vi "2039_hw Brake.vi"(2 "error in (no error)":errorcluster, 3 "CAN Talon SRX Ref":T1[](array[typedef])) -> (0 "error out":errorcluster, 1 "CAN Talon SRX Ref Out":T1[](array[typedef]))   [LabVIEW 2015]
uses:
  <vilib>/Rock Robotics/WPI/MotorControl/WPI_MotorControlDeviceRef.ctl
  <vilib>/Rock Robotics/WPI/MotorControl/WPI_MotorControlType.ctl
  <vilib>/Rock Robotics/SystemInterfaces/DIO/FPGA_DIOPWMChannel.ctl
  <vilib>/Rock Robotics/WPI/PWM/WPI_PWMDeadband.ctl
  <vilib>/Rock Robotics/WPI/CAN/Jaguar/SubVIs/WPI_CANJaguar_ControlMode.ctl
  <vilib>/Rock Robotics/WPI/CAN/TalonSRX/WPI_CANTalonSRX_APIControlMode.ctl
  <vilib>/Rock Robotics/WPI/CAN/TalonSRX/WPI_CANTalonSRX_BrakeOverride.ctl
  <vilib>/Rock Robotics/WPI/Utilities/WPI_GetSetVariantRefNum.vi
  <vilib>/Rock Robotics/WPI/RobotDrive/WPI_RobotDriveMecanumDrive_Cartesian.vi
  <vilib>/Rock Robotics/Network Tables/NT Write Numeric Array.vi
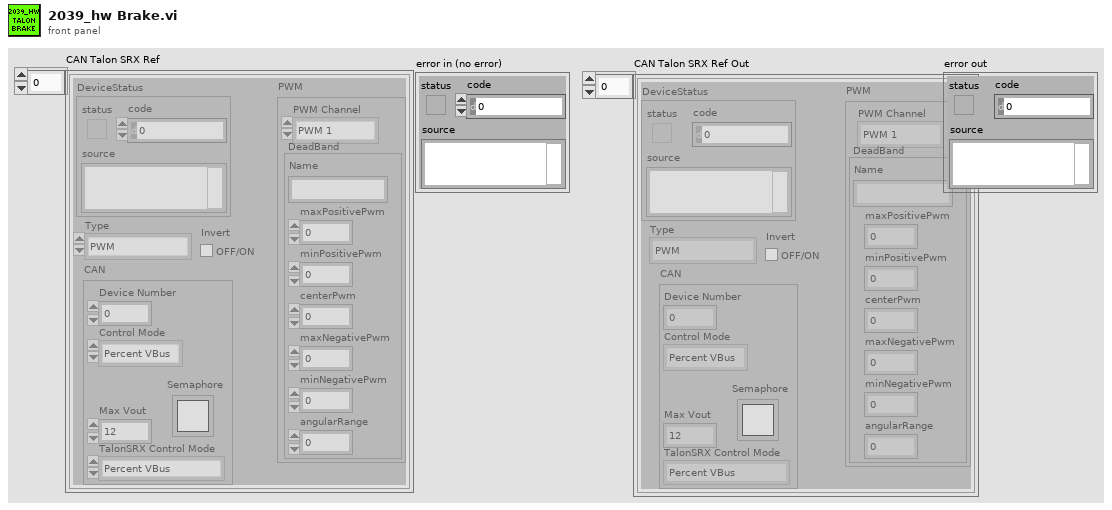
[diagram p1: front panel]
types:
  T1 = typedef "WPI_MotorControlDeviceRef.ctl" = cluster{"DeviceStatus":errorcluster, "Type":T2, "PWM":cluster{"PWM Channel":T3, "DeadBand":T4}, "CAN":cluster{"Device Number":u8, "Control Mode":T5, "Semaphore":T6, "Max Vout":dbl, "TalonSRX Control Mode":T7}, "Invert":bool}
  T2 = typedef "WPI_MotorControlType.ctl" = enum16{"PWM", "CAN", "CANTalonSRX"}
  T3 = typedef "FPGA_DIOPWMChannel.ctl" = enum8{"PWM 0", "PWM 1", "PWM 2", "PWM 3", "PWM 4", "PWM 5", "PWM 6", "PWM 7", "PWM 8", "PWM 9", "PWM MXP 0", "PWM MXP 1", "PWM MXP 2", "PWM MXP 3", "PWM MXP 4", "PWM MXP 5", "PWM MXP 6", "PWM MXP 7", "PWM MXP 8", "PWM MXP 9", "Invalid"}
  T4 = typedef "WPI_PWMDeadband.ctl" = cluster{"Name":string, "maxPositivePwm":i32, "minPositivePwm":i32, "centerPwm":i32, "maxNegativePwm":i32, "minNegativePwm":i32, "angularRange":u16}
  T5 = typedef "WPI_CANJaguar_ControlMode.ctl" = enum8{"Percent VBus", "Current", "Speed", "Position", "Voltage"}
  T6 = typedef "Semaphore RefNum" = refnum<k1>
  T7 = typedef "WPI_CANTalonSRX_APIControlMode.ctl" = enum8{"Percent VBus", "Speed", "Position", "Slave", "Unchanged / Invalid", "Voltage Compensation", "Current", "Motion Profile"}
  T8 = typedef "WPI_CANTalonSRX_BrakeOverride.ctl" = enum8{"No Override", "Override to Coast", "Override to Brake"}
  T9 = typedef "WPI_RobotDriveDevRef.ctl" = cluster{"DevStatus":errorcluster, "Motors[]":T1[], "Square Inputs":bool, "Max Output":dbl}
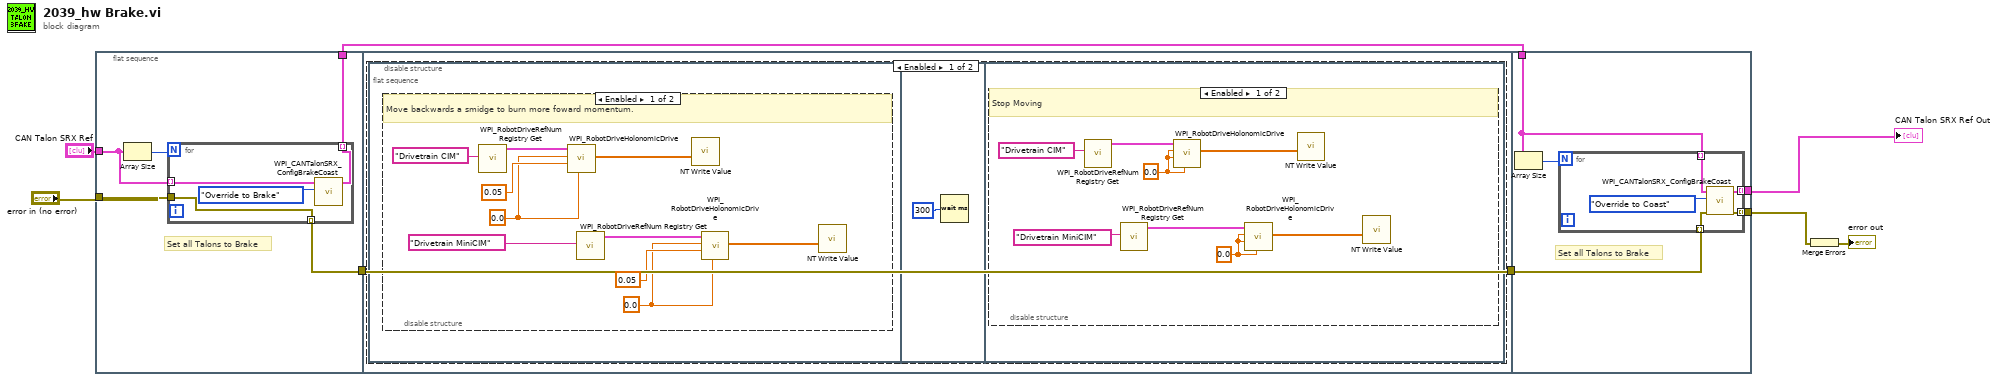
[diagram p0: block diagram]
diagram:
  n1 = flat-sequence {
    tunnel: "error in (no error)" -> [w12]
    tunnel: "CAN Talon SRX Ref" -> [w11]
    tunnel: [w10] -> w3
    tunnel: [w9] -> w5
    tunnel: w5 -> [w18]
    tunnel: [w18] -> w4
    tunnel: w4 -> [w41]
    tunnel: w3 -> [w40]
    tunnel: [w39] -> w2
    tunnel: [w38] -> w1
    frame #0 {
      # "Set all Talons to Brake"
      n2 = Array Size(array=w11) -> (size(s)=w13:i32)
      n3 = for {
        N: w13 -> [_]
        tunnel: w12 -> [w14]
        tunnel: w11 -> [w16] mode=indexing
        tunnel: [w15] -> w10 mode=indexing
        tunnel: [w14] -> w9 mode=indexing
        n4 = call <vilib>:"WPI_CANTalonSRX_ConfigBrakeCoast.vi"("Brake / Coast Mode"=WPI_CANTalonSRX_BrakeOverride."Override to Brake", "CAN Talon SRX Ref"=w16) -> ("CAN Talon SRX Ref"=w15:T1)  [unwired: 8 in, 1 out]
      }
    }
    frame #1 {
      n5 = disable-structure shown="Enabled" {
        frame Enabled {
          n6 = flat-sequence {
            frame #0 {
              n7 = disable-structure shown="Enabled" {
                frame Enabled {
                  w19 = 0.0
                  w20 = 0.0 ("X axis value")
                  # "Move backwards a smidge to burn more foward momentum."
                  n8 = call <vilib>:"WPI_RobotDriveRefNum Registry Get.vi"("refnum name"="Drivetrain CIM") -> ("RobotDriveDevRef"=w26:T9)  [unwired: 1 in, 9 out]
                  n9 = call-poly <vilib>:"WPI_RobotDriveHolonomicDrive.vi"("Rotation"=w19, "Y"=0.05, "X"=w19, "RobotDriveDevRef"=w26) -> ("Motor Values"=w27:dbl[])  [unwired: 5 in, 2 out]
                  n10 = call <vilib>:"WPI_RobotDriveRefNum Registry Get.vi"("refnum name"="Drivetrain MiniCIM") -> ("RobotDriveDevRef"=w23:T9)  [unwired: 1 in, 9 out]
                  n11 = call-poly <vilib>:"NT Write Value.vi"("Numeric Array"=w27) -> ()  [unwired: 10 in, 1 out]
                  n12 = call-poly <vilib>:"WPI_RobotDriveHolonomicDrive.vi"("Rotation"=w20, "Y"=0.05 ("X axis value"), "X"=w20, "RobotDriveDevRef"=w23) -> ("Motor Values"=w25:dbl[])  [unwired: 5 in, 2 out]
                  n13 = call-poly <vilib>:"NT Write Value.vi"("Numeric Array"=w25) -> ()  [unwired: 10 in, 1 out]
                }
                frame Disabled {
                }
              }
            }
            frame #1 {
              n14 = Wait (ms)(milliseconds to wait=300) -> ()  [unwired: 1 out]
            }
            frame #2 {
              n15 = disable-structure shown="Enabled" {
                frame Enabled {
                  w30 = 0.0
                  w31 = 0.0 ("X axis value")
                  # "Stop Moving"
                  n16 = call <vilib>:"WPI_RobotDriveRefNum Registry Get.vi"("refnum name"="Drivetrain CIM") -> ("RobotDriveDevRef"=w35:T9)  [unwired: 1 in, 9 out]
                  n17 = call <vilib>:"WPI_RobotDriveRefNum Registry Get.vi"("refnum name"="Drivetrain MiniCIM") -> ("RobotDriveDevRef"=w32:T9)  [unwired: 1 in, 9 out]
                  n18 = call-poly <vilib>:"WPI_RobotDriveHolonomicDrive.vi"("Rotation"=w30, "Y"=w30, "X"=w30, "RobotDriveDevRef"=w35) -> ("Motor Values"=w36:dbl[])  [unwired: 5 in, 2 out]
                  n19 = call-poly <vilib>:"WPI_RobotDriveHolonomicDrive.vi"("Rotation"=w31, "Y"=w31, "X"=w31, "RobotDriveDevRef"=w32) -> ("Motor Values"=w34:dbl[])  [unwired: 5 in, 2 out]
                  n20 = call-poly <vilib>:"NT Write Value.vi"("Numeric Array"=w36) -> ()  [unwired: 10 in, 1 out]
                  n21 = call-poly <vilib>:"NT Write Value.vi"("Numeric Array"=w34) -> ()  [unwired: 10 in, 1 out]
                }
                frame Disabled {
                }
              }
            }
          }
        }
        frame Disabled {
        }
      }
    }
    frame #2 {
      # "Set all Talons to Brake"
      n22 = Array Size(array=w40) -> (size(s)=w42:i32)
      n23 = for {
        N: w42 -> [_]
        tunnel: w41 -> [w46] mode=indexing
        tunnel: w40 -> [w45] mode=indexing
        tunnel: [w44] -> w39 mode=indexing
        tunnel: [w43] -> w38 mode=indexing
        n24 = call <vilib>:"WPI_CANTalonSRX_ConfigBrakeCoast.vi"("error in (no error)"=w46, "Brake / Coast Mode"=WPI_CANTalonSRX_BrakeOverride."Override to Coast", "CAN Talon SRX Ref"=w45) -> ("error out"=w43:errorcluster, "CAN Talon SRX Ref"=w44:T1)  [unwired: 7 in]
      }
    }
  }
  n25 = Merge Errors(w1) -> (→"error out":errorcluster)
  "CAN Talon SRX Ref Out" <- w2
